vi "Method.vi"(8 "error in (no error)":errorcluster, 11 "Child 2 in":refnum<class "Child 2.lvclass">) -> (0 "error out":errorcluster, 2 "Output":string, 3 "Child 2 out":refnum<class "Child 2.lvclass">)   [LabVIEW 2017, in "Child 2.lvclass"]
uses:
  Child 2.lvclass
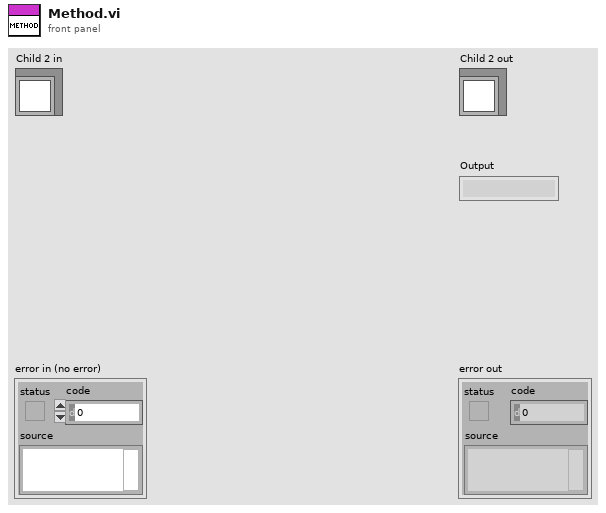
[diagram p1: front panel]
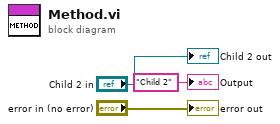
[diagram p0: block diagram]
diagram:
  "error out" <- "error in (no error)"
  "Child 2 out" <- "Child 2 in"
  "Output" <- "Child 2" ("Output")
